vi "Check Measure complete.vi"(0 "Measurements":T1[](array[typedef]), 5 "Instrument handle":refnum<k15>[](array[refnum]), 7 "Channel Number":string[](array[string]), 11 "error in (no error)":errorcluster) -> (6 "Measure complete?":bool[](array[boolean]), 15 "error out":errorcluster)   [LabVIEW 2024, in "devicePowerSequencingModuleCoreLogic.lvlib"]
uses:
  devicePowerSequencingModuleCoreLogic.lvlib
  controls/Voltage and Current Measurements.ctl
panel:
  in  "Pin Name":string[](array[string])
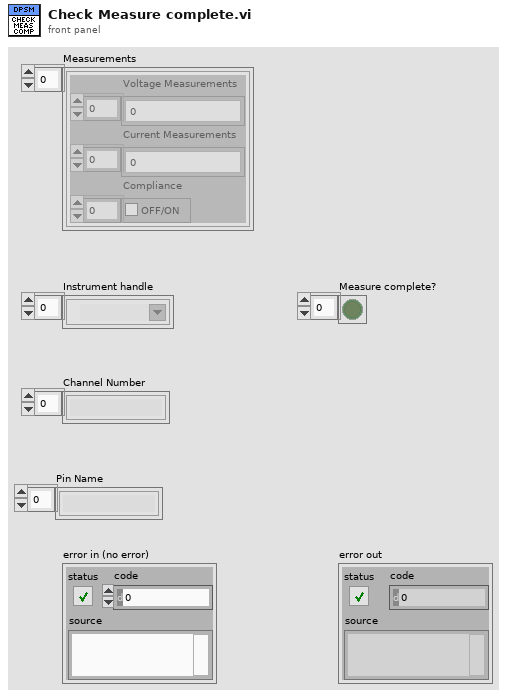
[diagram p1: front panel]
types:
  T1 = typedef "devicePowerSequencingModuleCoreLogic.lvlib/Voltage and Current Measurements.ctl" = cluster{"Voltage Measurements":dbl[], "Current Measurements":dbl[], "Compliance":bool[]}
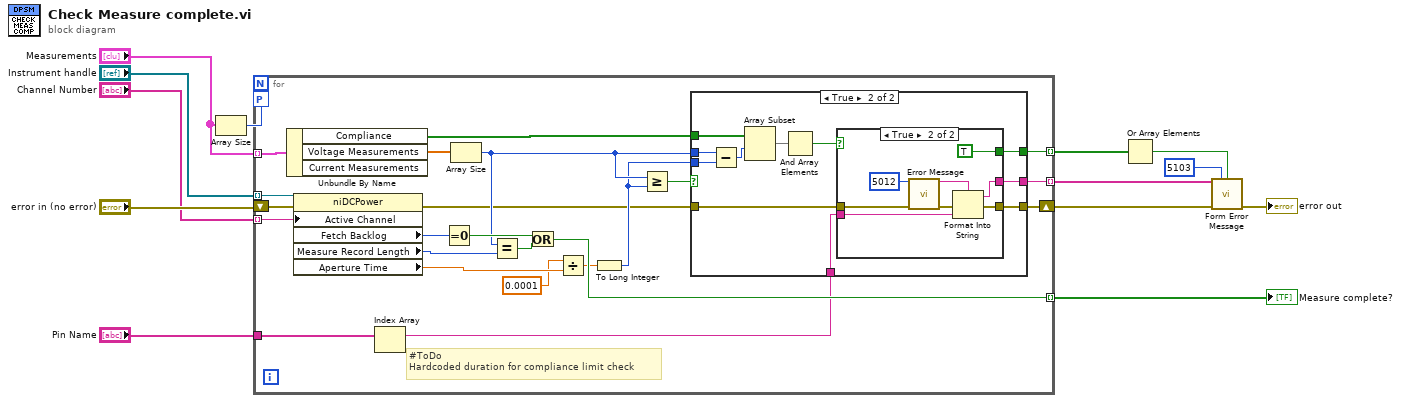
[diagram p0: block diagram]
diagram:
  n1 = Array Size(array="Measurements") -> (size(s)=w12:i32)
  n2 = for {
    tunnel: "Instrument handle" -> [w35] mode=indexing
    tunnel: "Channel Number" -> [w34] mode=indexing
    shift-right: [w18] -> w3
    shift-left: "error in (no error)" -> [w36]
    tunnel: [w31] -> w1 mode=indexing
    tunnel: "Measurements" -> [w30] mode=indexing
    workers-P: w12 -> [_]
    tunnel: "Pin Name" -> [w17]
    tunnel: [w16] -> w5 mode=indexing
    tunnel: [w15] -> w4 mode=indexing
    # "#ToDo \nHardcoded duration for compliance limit check"
    n3 = Unbundle By Name(w30) -> ("Compliance"=w26:bool[], "Voltage Measurements"=w27:dbl[])  [unwired: 1 out]
    n4 = property class="niDCPower"(reference=w35, error in=w36, "Active Channel"=w34) -> (error out=w19:errorcluster, "Fetch Backlog"=w33:i32, "Measure Record Length"=w28:i32, "Aperture Time"=w25:dbl)  [unwired: 1 out]
    n5 = Index Array(array=w17) -> (element=w14:string)  [unwired: 1 in]
    n6 = Equal To 0?(x=w33) -> (x = 0?=w32:bool)
    n7 = Array Size(array=w27) -> (size(s)=w23:i32)
    n8 = Equal?(x=w23, y=w28) -> (x = y?=w29:bool)
    n9 = Or(x=w32, y=w29) -> (x .or. y?=w31:bool)
    n10 = Divide(x=0.0001, y=w25) -> (x/y=w22:dbl)
    n11 = To Long Integer(number=w22) -> (32bit integer=w20:i32)
    n12 = Greater Or Equal?(x=w23, y=w20) -> (x >= y?=w21:bool)
    n13 = case shown="True" w21 {
      tunnel: w26 -> [_ w47]
      tunnel: w23 -> [_ w45]
      tunnel: w20 -> [_ w44]
      tunnel: w19 -> [w37 w43]
      tunnel: [w37 w41] -> w18
      tunnel: w14 -> [_ w42]
      tunnel: [_ w40] -> w16
      tunnel: [_ w39] -> w15
      frame False {
        # "Don't check for compliance"
      }
      frame True {
        n14 = Subtract(x=w45, y=w44) -> (x-y=w48:i32)
        n15 = Array Subset(array=w47, index=w48) -> (w46:bool[])  [unwired: 1 in]
        n16 = And Array Elements(Boolean array=w46) -> (logical AND=w38:bool)
        n17 = case shown="True" w38 {
          tunnel: w43 -> [w49 w57]
          tunnel: [w49 w52] -> w41
          tunnel: [_ w54] -> w39
          tunnel: [_ TRUE] -> w40
          tunnel: w42 -> [_ w51]
          frame False {
            # "Check Passed"
          }
          frame True {
            n18 = call "Error Message.vi"("Error Code"=5012, "error in (no error)"=w57) -> ("Error Message"=w50:string, "error out"=w53:errorcluster)  [unwired: 11 in, 1 out]
            n19 = Format Into String(format string=w50, error in=w53, w51) -> (resulting string=w54:string, error out=w52:errorcluster)  [unwired: 1 in]
          }
        }
      }
    }
  }
  "Measure complete?" <- w1
  n20 = Or Array Elements(Boolean array=w5) -> (logical OR=w6:bool)
  n21 = call "Form Error Message.vi"("Error Message"=w4, "error code (0)"=5103, "Error?"=w6, "error in (no error)"=w3) -> ("error out"=→"error out":errorcluster)  [unwired: 11 in]
